vi "Get SMO PGSQL Log Paths.vi"(5 "getAll Cluster":variant, 7 "Default Paths":string, 8 "error in (no error)":errorcluster, 11 "Instrument in":refnum<class "Instrument.lvclass">) -> (0 "error out":errorcluster, 2 "Paths":string, 3 "Instrument out":refnum<class "Instrument.lvclass">)   [LabVIEW 2019, in "Instrument.lvclass"]
uses:
  Instrument.lvclass
  Instrument.lvclass/Instrument.ctl
  <userlib>/LevyLab/LV-Data/LV-Data.PG/LV-Data.PGSQL.lvclass
  <userlib>/LevyLab/LV-Data/LV-Data.PG/API/Write Variable (one-row).vi
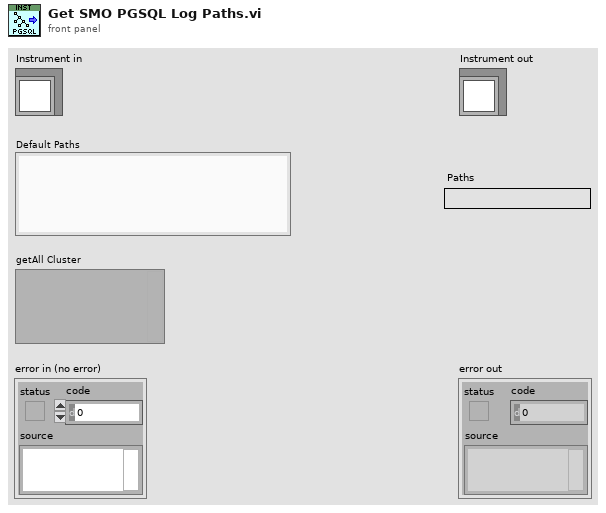
[diagram p1: front panel]
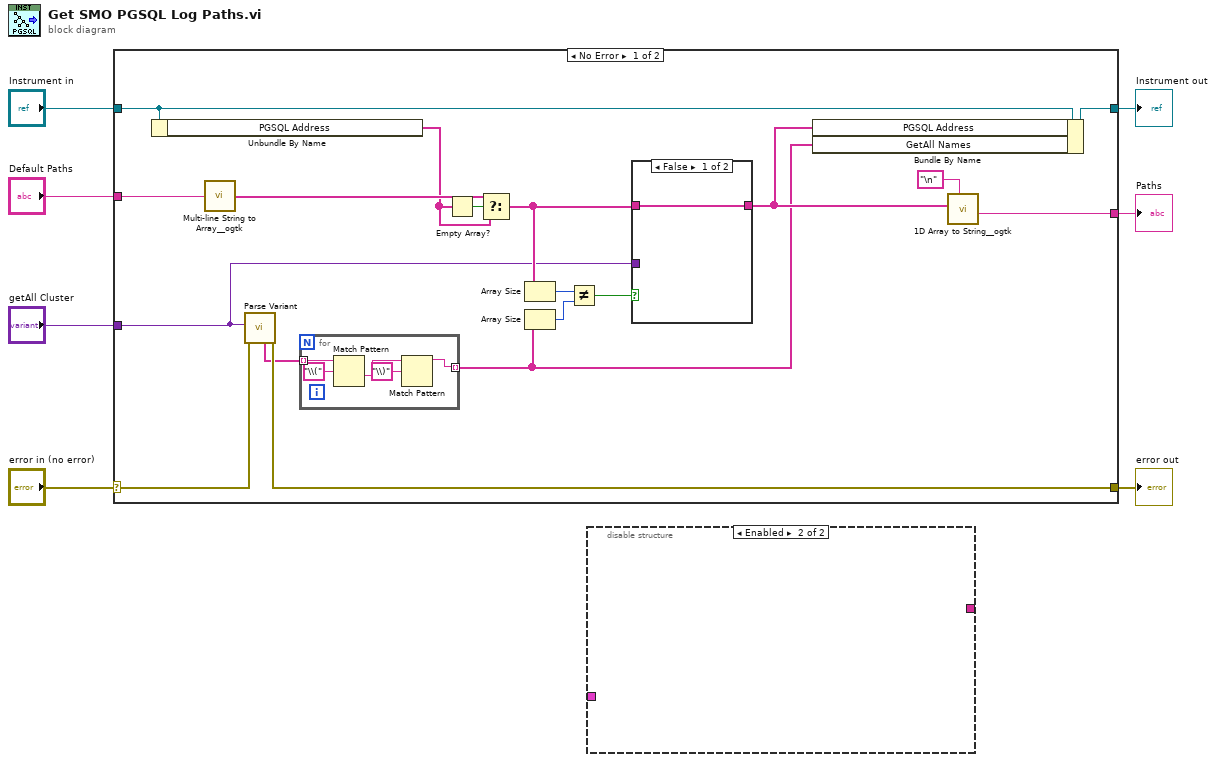
[diagram p0: block diagram]
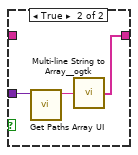
[diagram p2: hidden frame]
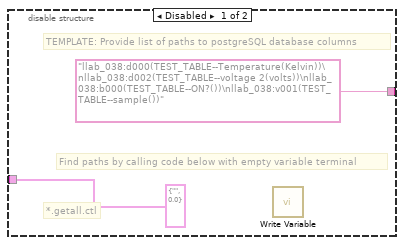
[diagram p4: hidden frame]
diagram:
  n1 = case shown="No Error" "error in (no error)" {
    selector: "error in (no error)" -> [w11 w36]
    tunnel: [w10 w36] -> w6
    tunnel: [w24 w35] -> w4
    tunnel: "Instrument in" -> [w25 w35]
    tunnel: "Default Paths" -> [w22 _]
    tunnel: [w20 _] -> w2
    tunnel: "getAll Cluster" -> [w9 _]
    frame No Error {
      n2 = Unbundle By Name(w25) -> ("PGSQL Address"=w18:string[])
      n3 = call <userlib>:"Multi-line String to Array__ogtk.vi"("string"=w22) -> ("lines"=w19:string[])
      n4 = call <userlib>:"Parse Variant.vi"("error in"=w11, "Data"=w9) -> ("error out"=w10:errorcluster, "Type (Name)"=w8:string[])  [unwired: 5 in, 3 out]
      n5 = for {
        tunnel: w8 -> [w29] mode=indexing
        tunnel: [w26] -> w12 mode=indexing
        n6 = Match Pattern(string=w29, regular expression="\\(") -> (after substring=w27:string)  [unwired: 1 in, 3 out]
        n7 = Match Pattern(string=w27, regular expression="\\)") -> (before substring=w26:string)  [unwired: 1 in, 3 out]
      }
      n8 = Empty Array?(array=w18) -> (empty?=w23:bool)
      n9 = Select(t=w19, s=w23, f=w18) -> (s? t:f=w15:string[])
      n10 = Array Size(array=w15) -> (size(s)=w13:i32)
      n11 = Array Size(array=w12) -> (size(s)=w17:i32)
      n12 = Not Equal?(x=w13, y=w17) -> (x != y?=w16:bool)
      n13 = case shown="False" w16 {
        tunnel: w9 -> [_ w34]
        tunnel: [w31 w32] -> w14
        tunnel: w15 -> [w31 _]
        frame False {
        }
        frame True {
          n14 = call <userlib>:"Get Paths Array UI.vi"("Data"=w34) -> ("selected_paths"=w33:string)  [unwired: 9 in, 1 out]
          n15 = call <userlib>:"Multi-line String to Array__ogtk.vi"("string"=w33) -> ("lines"=w32:string[])
        }
      }
      n16 = Bundle By Name(cluster=w25, "PGSQL Address"=w14, "GetAll Names"=w12) -> (w24:refnum<class "Instrument.lvclass">)
      n17 = call <userlib>:"1D Array to String__ogtk.vi"("delimiter (Tab)"="\n", "Array of Strings"=w14) -> ("delimited string"=w20:string)  [unwired: 9 in]
    }
    frame Error {
    }
  }
  "error out" <- w6
  "Instrument out" <- w4
  "Paths" <- w2
  n18 = disable-structure shown="Enabled" {
    disable-tunnel: ["llab_038:d000(TEST_TABLE--Temperature(Kelvin))\nllab_038:d002(TEST_TABLE--voltage 2(volts))\nllab_038:b000(TEST_TABLE--ON?())\nllab_038:v001(TEST_TABLE--sample())" ("Paths") _] -> _
    disable-tunnel: [cluster{string, dbl} {"", 0.0} _] -> _
    frame Disabled {
      # "Find paths by calling code below with empty variable terminal"
      # "*.getall.ctl"
      # "TEMPLATE: Provide list of paths to postgreSQL database columns"
      n19 = call-poly <userlib>:"Write Variable.vi"() -> ()  [unwired: 8 in, 4 out]
    }
    frame Enabled {
    }
  }
